vi "rs3 Advanced set Color control3.vi"(8 "error in (no error)":errorcluster, 10 "ST Color Control":T1, 11 "device in":u64) -> (0 "error out":errorcluster, 1 "error":u64, 3 "Dev out":u64)   [LabVIEW 2018, in "libRealSense3.lvlib"]
doc: "This sets some register that affect the depth calculations"
uses:
  libRealSense3.lvlib
  realsense2.dll
panel:
  # "RS3 Adv. Set Color Control 2"
  # "(C) 2017 Intel Corp.,  AGJ"
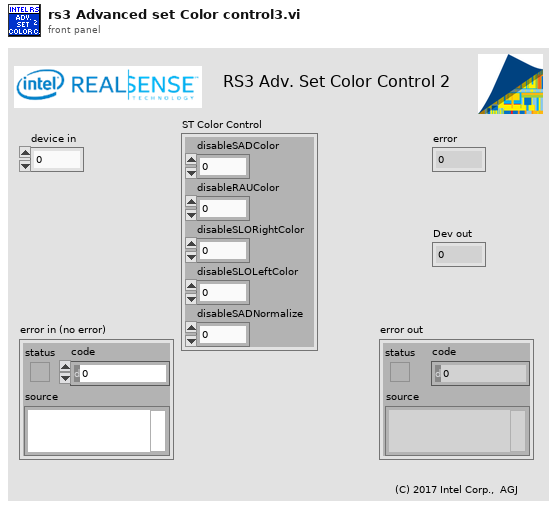
[diagram p1: front panel]
types:
  T1 = cluster{"disableSADColor":u32, "disableRAUColor":u32, "disableSLORightColor":u32, "disableSLOLeftColor":u32, "disableSADNormalize":u32}
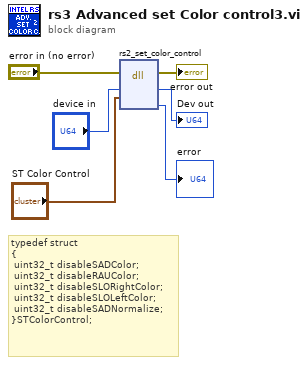
[diagram p0: block diagram]
diagram:
  # "typedef struct\n{\n\tuint32_t disableSADColor;\n\tuint32_t disableRAUColor;\n\tuint32_t disableSLORightColor;\n\tuint32_t disableSLOLeftColor;\n\tuint32_t disableSADNormalize;\n}STColorControl;"
  n1 = dll-call lib="C:/Users/aaron.jencks/Documents/GitHub/emerson_seed_object_detection/LabVIEW/Projects/Paul's Video Viewer/Classes/Realsense Cam/realsense_wrapper_api/realsense2.dll" fn="rs2_set_color_control"(error in="error in (no error)", "device"="device in", "ST Color Control"="ST Color Control") -> (error out=→"error out":errorcluster, "device"=→"Dev out":u64, "error"=→"error":u64)  [unwired: 5 in, 1 out]
